vi "Quadratic Roots.vi"() -> ()   [LabVIEW 2025]
panel:
  out "Root 2":dbl
  out "Root 1":dbl
  in  "C":dbl
  in  "B":dbl
  in  "A":dbl
  # "ME 235: Design of Microprocessor Based Mechanical Systems"
  # "Lab 1 - Quadratic Roots"
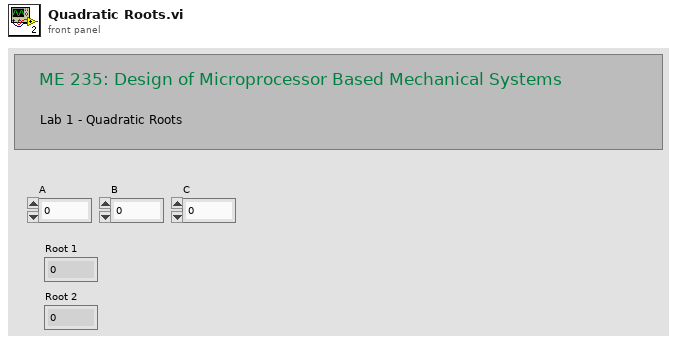
[diagram p1: front panel]
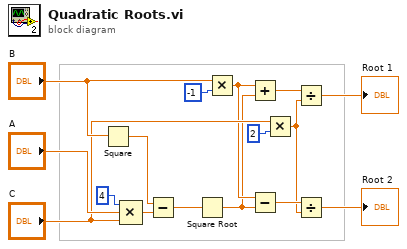
[diagram p0: block diagram]
diagram:
  n1 = Square(x="B") -> (x^2=w4:dbl)
  n2 = Compound Arithmetic op=MULTIPLY(4, "A", "C") -> (w3:dbl)
  n3 = Subtract(x=w4, y=w3) -> (x-y=w5:dbl)
  n4 = Square Root(x=w5) -> (sqrt(x)=w1:dbl)
  n5 = Multiply(x="B", y=-1) -> (x*y=w2:dbl)
  n6 = Add(x=w2, y=w1) -> (x+y=w13:dbl)
  n7 = Subtract(x=w2, y=w1) -> (x-y=w12:dbl)
  n8 = Multiply(x="C", y=2) -> (x*y=w11:dbl)
  n9 = Divide(x=w13, y=w11) -> (x/y=→"Root 1":dbl)
  n10 = Divide(x=w12, y=w11) -> (x/y=→"Root 2":dbl)
